vi "Transport Server.vi"   [LabVIEW 2019, in "Inst.Transport.lvclass"]
uses:
  Inst.Transport/Inst.Transport.lvclass
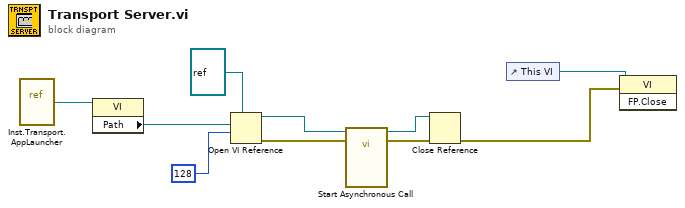
[diagram p0: block diagram]
diagram:
  n1 = vi-ref "Inst.Transport.AppLauncher.vi"() -> (w3:refnum<vi>)
  n2 = property class="VI"(reference=w3) -> ("Path"=w4:path)  [unwired: 1 in, 2 out]
  n3 = Open VI Reference(type specifier VI Refnum (for type only)=refnum<vi> refnum, vi path=w4, options=128) -> (vi reference=w2:refnum<vi>, error out=w10:errorcluster)  [unwired: 3 in]
  n4 = call-by-ref "Start Asynchronous Call"(reference=w2, error in=w10) -> (reference out=w8:refnum<vi>, error out=w9:errorcluster)  [unwired: 11 in, 1 out]
  n5 = Close Reference(reference=w8, error in (no error)=w9) -> (error out=w6:errorcluster)
  n6 = control-ref of="This VI"() -> (w7:refnum<vi>)
  n7 = invoke class="VI" method="FP.Close"(reference=w7, error in=w6) -> ()  [unwired: 1 in, 3 out]
